vi "MAR05.vi"() -> ()   [LabVIEW 2020]
panel:
  out "new picture 2":picture
  out "new picture":picture
  out "lowercase file extension":string
  in  "File Path":path
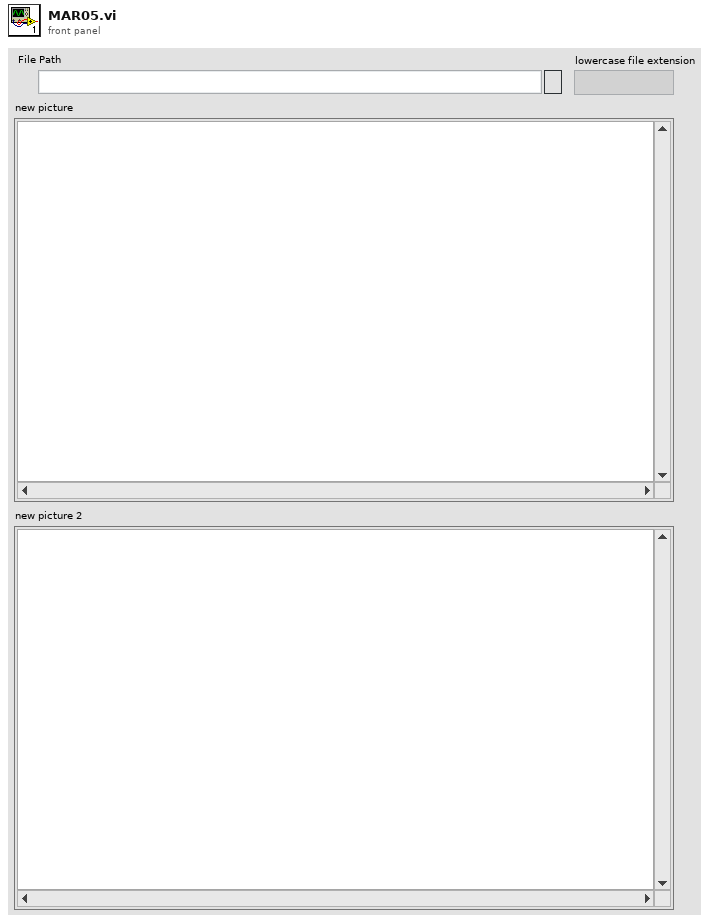
[diagram p1: front panel]
types:
  T1 = typedef "imagedata.ctl" = cluster{"image type":i32, "image depth":i32, "image":u8[], "mask":u8[], "colors":u32[], "Rectangle":cluster{"left":i16, "top":i16, "right":i16, "bottom":i16}}
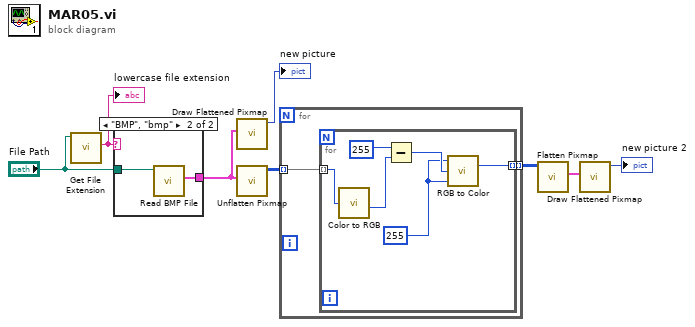
[diagram p0: block diagram]
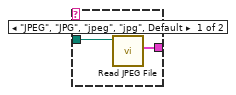
[diagram p2: hidden frame]
diagram:
  n1 = call <vilib>:"Get File Extension.vi"("file"="File Path") -> ("lowercase file extension"=w8:string)  [unwired: 6 in, 4 out]
  "lowercase file extension" <- w8
  n2 = case shown="\"BMP\", \"bmp\"" w8 {
    tunnel: "File Path" -> [w10 w12]
    tunnel: [w9 w11] -> w5
    frame "JPEG", "JPG", "jpeg", "jpg", Default {
      n3 = call <vilib>:"Read JPEG File.vi"("path to JPEG file"=w10) -> ("image data"=w9:T1)  [unwired: 8 in, 2 out]
    }
    frame "BMP", "bmp" {
      n4 = call <vilib>:"Read BMP File.vi"("path to BMP file"=w12) -> ("image data"=w11:T1)  [unwired: 8 in, 2 out]
    }
  }
  n5 = call <vilib>:"Draw Flattened Pixmap.vi"("image data"=w5) -> ("new picture"=→"new picture":picture)  [unwired: 8 in]
  n6 = call <vilib>:"Unflatten Pixmap.vi"("image data"=w5) -> ("24-bit pixmap"=w4:u32[][])  [unwired: 4 in, 6 out]
  n7 = for {
    tunnel: w4 -> [w14] mode=indexing
    tunnel: [w13] -> w3 mode=indexing
    n8 = for {
      tunnel: w14 -> [w20] mode=indexing
      tunnel: [w19] -> w13 mode=indexing
      w15 = u8 255 ("R")
      n9 = call <vilib>:"Color to RGB.vi"("Color"=w20) -> ("G"=w17:u8)  [unwired: 3 out]
      n10 = Subtract(x=u8 255 ("R"), y=w17) -> (x-y=w16:u8)
      n11 = call <vilib>:"RGB to Color.vi"("B"=w15, "G"=w16, "R"=w15) -> ("Color"=w19:u32)
    }
  }
  n12 = call <vilib>:"Flatten Pixmap.vi"("24-bit pixmap"=w3) -> ("image data"=w1:T1)  [unwired: 10 in]
  n13 = call <vilib>:"Draw Flattened Pixmap.vi"("image data"=w1) -> ("new picture"=→"new picture 2":picture)  [unwired: 8 in]
